vi "Add AOI to list.vi"(1 "AOI to add":u16[](array[numeric])) -> (0 "Number of AOIs":i32)   [LabVIEW 2016]
doc: "Adds a new AOI to the global AOI list."
uses:
  AOI List Globals.vi
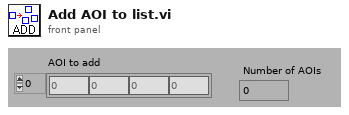
[diagram p1: front panel]
types:
  T1 = cluster{"AOI to add[0]":u16, "AOI to add[1]":u16, "AOI to add[2]":u16, "AOI to add[3]":u16}
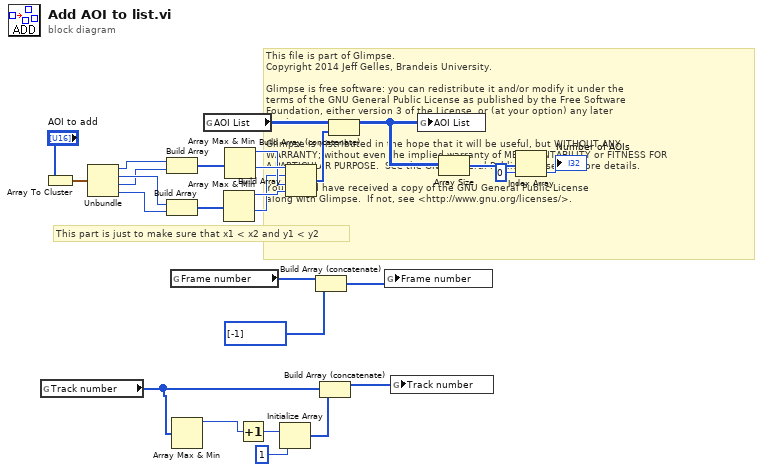
[diagram p0: block diagram]
diagram:
  # "This file is part of Glimpse. \nCopyright 2014 Jeff Gelles, Brandeis University.    \n\nGlimpse is free software: you can redistribute it and/or modify it under the \nterms of the GNU General Public License as published by the Free Software \nFoundation, either version 3 of the License, or (at your option) any later \nversion.\n\nGlimpse is distributed in the hope that it will be useful, but WITHOUT ANY \nWARRANTY; without even the implied warranty of MERCHANTABILITY or FITNESS FOR \nA PARTICULAR PURPOSE.  See the GNU General Public License for more details.\n\nYou should have received a copy of the GNU General Public License\nalong with Glimpse.  If not, see <http://www.gnu.org/licenses/>."
  # "This part is just to make sure that x1 < x2 and y1 < y2"
  n1 = global read "AOI List Globals.vi" "Track number"() -> (w5:u16[])
  n2 = Array To Cluster(array="AOI to add") -> (cluster=w21:T1)
  n3 = Unbundle(w21) -> ("AOI to add[0]"=w20:u16, "AOI to add[1]"=w19:u16, "AOI to add[2]"=w18:u16, "AOI to add[3]"=w17:u16)
  n4 = Build Array(w20, w18) -> (w16:u16[])
  n5 = Build Array(w19, w17) -> (w15:u16[])
  n6 = global read "AOI List Globals.vi" "Frame number"() -> (w8:i32[])
  n7 = Array Max & Min(array=w5) -> (max value=w4:u16)  [unwired: 3 out]
  n8 = global read "AOI List Globals.vi" "AOI List"() -> (w27:u16[][])
  n9 = Array Max & Min(array=w15) -> (max value=w12:u16, min value=w11:u16)  [unwired: 2 out]
  n10 = Array Max & Min(array=w16) -> (max value=w13:u16, min value=w14:u16)  [unwired: 2 out]
  n11 = Increment(x=w4) -> (x+1=w3:u16)
  n12 = Initialize Array(w3, 1 ("dimension size")) -> (w1:u16[])
  n13 = Build Array(w14, w11, w13, w12) -> (w10:u16[])
  n14 = Build Array (concatenate)(w8, i32[] [-1] ("array")) -> (w9:i32[])
  n15 = Build Array (concatenate)(w5, w1) -> (w6:u16[])
  n16 = Build Array (concatenate)(w27, w10) -> (w26:u16[][])
  n17 = global write "AOI List Globals.vi" "Frame number"(w9) -> ()
  n18 = global write "AOI List Globals.vi" "Track number"(w6) -> ()
  n19 = global write "AOI List Globals.vi" "AOI List"(w26) -> ()
  n20 = Array Size(array=w26) -> (size(s)=w24:i32[])
  n21 = Index Array(array=w24, index=0) -> (element=→"Number of AOIs":i32)
